vi "Get Type Cast Test Settings.vi"(8 "Error In":errorcluster, 11 "Data Channel Ref In":T1 format="%.0x") -> (0 "Error out":errorcluster, 2 "Data Channel Settings":T2, 3 "Data Channel Ref Out":T1=18446744073709551615 format="%.0x")   [LabVIEW 2020, in "Instrument Addon Scripting API Channels Unit Tests.lvclass"]
uses:
  Instrument Addon Scripting API Channels Unit Tests.lvclass
  <vilib>/NI VeriStand/Custom Device API/Custom Device Item Ref.ctl
  APIs/Scripting API/TypeDefs/Array Type Cast Settings.ctl
  APIs/Scripting API/TypeDefs/Array Element.ctl
  Addon/Addon Shared/Types/Type Cast Type.ctl
  Addon/Addon Shared/Types/Endian.ctl
  <vilib>/NI VeriStand/Custom Device API/Get Item Property (String).vi
  <vilib>/NI VeriStand/Custom Device API/Get Item Property (U16).vi
  <vilib>/NI VeriStand/Custom Device API/Custom Device API.lvlib
  Addon/Addon Shared/Instrument Addon Shared.lvlib
  APIs/Scripting API/Instrument Addon Scripting API.lvlib
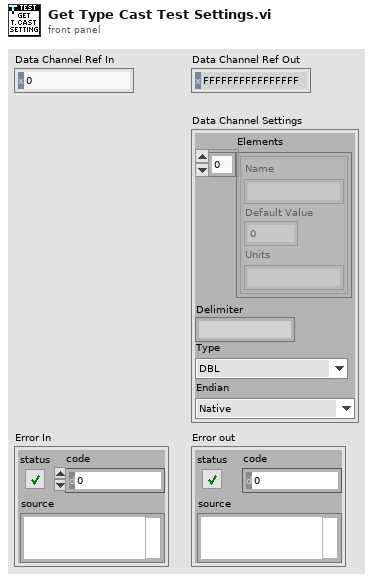
[diagram p1: front panel]
types:
  T1 = typedef "Custom Device API.lvlib/Custom Device Item Ref.ctl" = u64
  T2 = typedef "Instrument Addon Scripting API.lvlib/Array Type Cast Settings.ctl" = cluster{"Elements":T3[], "Delimiter":string, "Type":T4, "Endian":T5}
  T3 = typedef "Instrument Addon Scripting API.lvlib/Array Element.ctl" = cluster{"Name":string, "Default Value":dbl, "Units":string}
  T4 = typedef "Instrument Addon Shared.lvlib/Type Cast Type.ctl" = enum16{"DBL", "SGL", "U64", "U32", "U16", "U8", "I64", "I32", "I16", "I8"}
  T5 = typedef "Instrument Addon Shared.lvlib/Endian.ctl" = enum16{"Native", "Little", "Big"}
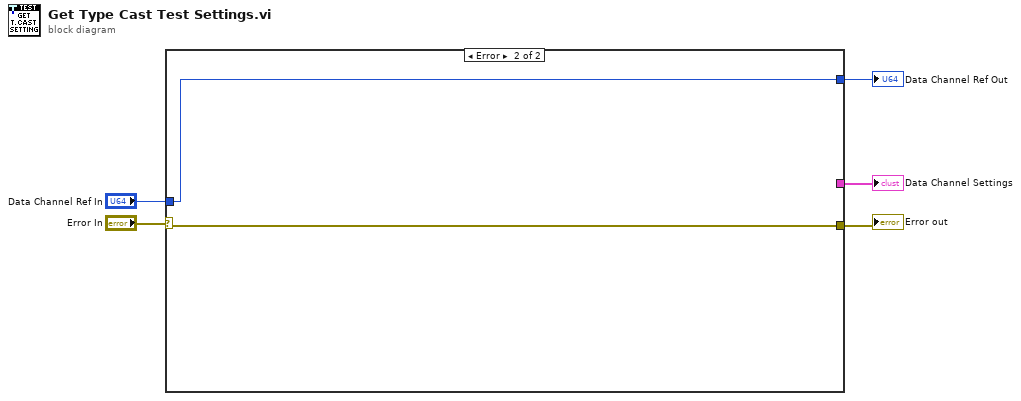
[diagram p0: block diagram]
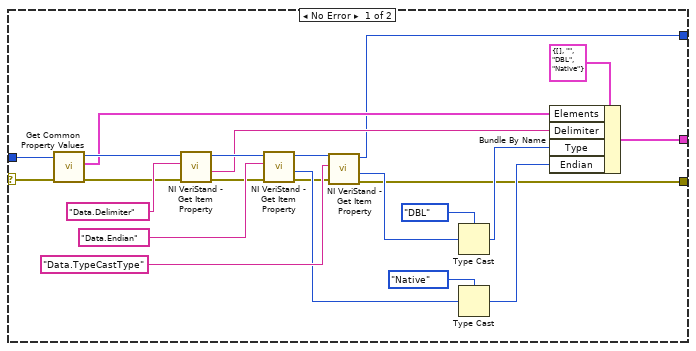
[diagram p2: hidden frame]
diagram:
  n1 = case shown="Error" "Error In" {
    selector: "Error In" -> [w8 w29]
    tunnel: [w28 _] -> w5
    tunnel: [w12 w29] -> w4
    tunnel: "Data Channel Ref In" -> [w10 w30]
    tunnel: [w6 w30] -> w1
    frame No Error {
      n2 = call "Get Common Property Values.vi"("Error In"=w8, "Data Channel  Ref in"=w10) -> ("error out"=w11:errorcluster, "Array Out"=w7:T3[], "Data Channel Ref Out"=w9:u64)  [unwired: 7 in]
      n3 = call-poly <vilib>:"NI VeriStand - Get Item Property.vi"("error in (no error)"=w11, "Property Name"="Data.Delimiter", "Item Ref in"=w9) -> ("error out"=w18:errorcluster, "Value"=w15:string, "Item Ref out"=w20:T1)  [unwired: 5 in, 1 out]
      n4 = call-poly <vilib>:"NI VeriStand - Get Item Property.vi"("error in (no error)"=w18, "Property Name"="Data.Endian", "Item Ref in"=w20) -> ("error out"=w19:errorcluster, "Value"=w22:u16, "Item Ref out"=w21:T1)  [unwired: 5 in, 1 out]
      n5 = call-poly <vilib>:"NI VeriStand - Get Item Property.vi"("error in (no error)"=w19, "Property Name"="Data.TypeCastType", "Item Ref in"=w21) -> ("error out"=w12:errorcluster, "Value"=w16:u16, "Item Ref out"=w6:T1)  [unwired: 5 in, 1 out]
      n6 = Type Cast(type=Type_Cast_Type."DBL" ("Type"), x=w16) -> (*(type *) &x=w17:T4)
      n7 = Type Cast(type=Endian."Native" ("Endian"), x=w22) -> (*(type *) &x=w23:T5)
      n8 = Bundle By Name(cluster=T2 {"Elements"=[], "Delimiter"="", "Type"=enum."DBL", "Endian"=enum."Native"} ("Settings"), "Elements"=w7, "Delimiter"=w15, "Type"=w17, "Endian"=w23) -> (w28:T2)
    }
    frame Error {
    }
  }
  "Data Channel Settings" <- w5
  "Error out" <- w4
  "Data Channel Ref Out" <- w1
